vi "testEscapeCharsInAttributes.vi"(8 "error in (no error)":errorcluster, 11 "reference in":refnum<class "EasyXMLTest.lvclass">) -> (0 "error out":errorcluster, 3 "reference in":refnum<class "EasyXMLTest.lvclass">)   [LabVIEW 2011, in "EasyXMLTest.lvclass"]
uses:
  EasyXMLTest.lvclass
panel:
  out "Generated XML String":string
  out "Escape Chars":T1
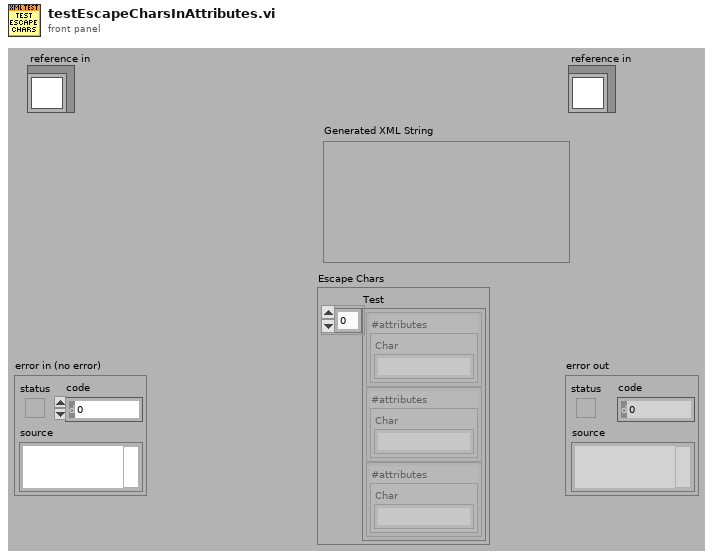
[diagram p1: front panel]
types:
  T1 = cluster{"Test":cluster{"#attributes":cluster{"Char":string}}[]}
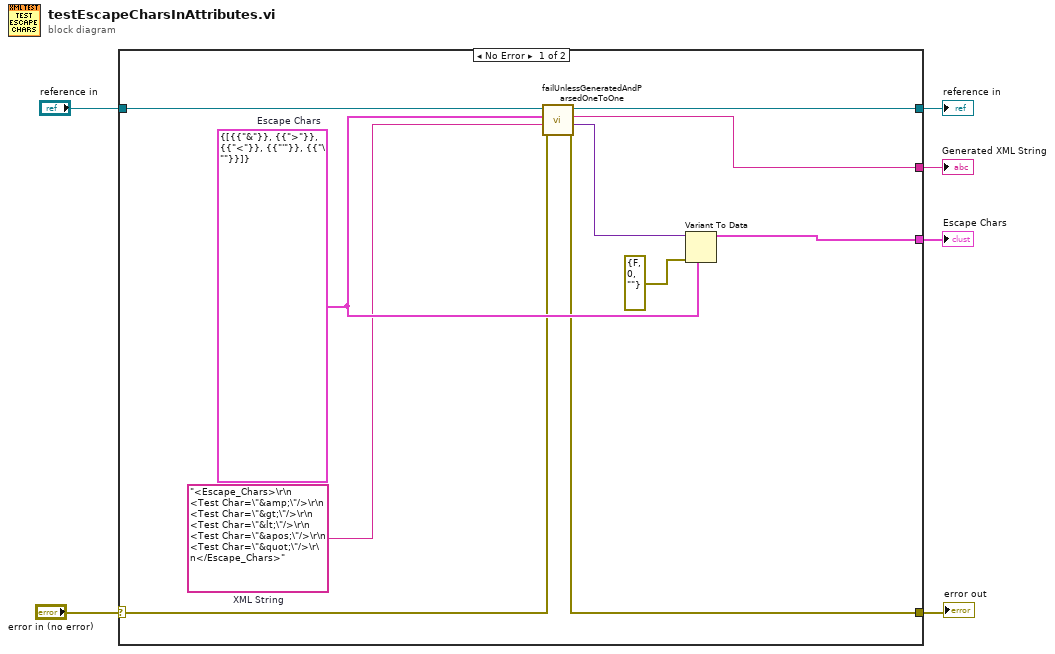
[diagram p0: block diagram]
diagram:
  n1 = case shown="No Error" "error in (no error)" {
    selector: "error in (no error)" -> [w10 w18]
    tunnel: [w9 w18] -> w5
    tunnel: [w13 w17] -> w3
    tunnel: "reference in" -> [w14 w17]
    tunnel: [w8 _] -> w2
    tunnel: [w16 _] -> w1
    frame No Error {
      w12 = T1 {"Test"=[{"#attributes"={"Char"="&"}}, {"#attributes"={"Char"=">"}}, {"#attributes"={"Char"="<"}}, {"#attributes"={"Char"="'"}}, {"#attributes"={"Char"="\""}}]}  # Escape Chars
      w11 = "<Escape_Chars>\r\n  <Test Char=\"&amp;\"/>\r\n  <Test Char=\"&gt;\"/>\r\n  <Test Char=\"&lt;\"/>\r\n  <Test Char=\"&apos;\"/>\r\n  <Test Char=\"&quot;\"/>\r\n</Escape_Chars>"  # XML String
      n2 = call "failUnlessGeneratedAndParsedOneToOne.vi"("error in"=w10, "XML String"=w11, "Data"=w12, "EasyXMLTest in"=w14) -> ("error out"=w9:errorcluster, "Produced Data"=w7:variant, "Generated XML String"=w8:string, "EasyXMLTest out"=w13:refnum<class "EasyXMLTest.lvclass">)  [unwired: 4 in]
      n3 = Variant To Data(error in=errorcluster {"status"=FALSE, "code"=0, "source"=""}, type=w12, Variant=w7) -> (data=w16:T1)  [unwired: 1 out]
    }
    frame Error {
    }
  }
  "error out" <- w5
  "reference in" <- w3
  "Generated XML String" <- w2
  "Escape Chars" <- w1
